vi "Valid waveforms Write.vi"(4 "error in (no error)":errorcluster, 5 "Value":T1[](array[typedef]), 6 "Container State":T4, 7 "Display State In":T2) -> (0 "error out":errorcluster, 3 "Display State Out":T2)   [LabVIEW 2020, in "Waveform (G3).xctl"]
uses:
  Waveform (G3).xctl
  <vilib>/_xctls/Container State.ctl
  State.ctl
  Utility VIs/Controls/KRing/KRing.xctl
  Tone (G3)/Tone (G3).xctl
  Noise (G3)/Noise (G3).xctl
  Noise (G3)/Noise (G3) - Persistent.ctl
  Waveform VIs/Waveform Enum (V3).ctl
  <vilib>/_xctls/XControlSupport.lvlib
panel:
  in  "Waveform":T1
  # "Replace the Value Control below with a Control of desired type.\nDo not remove this Control or the others from the connector pane.\nDo not change the connector pane pattern.\nThe Value control should always be the third terminal from top on the input side in the connector pane."
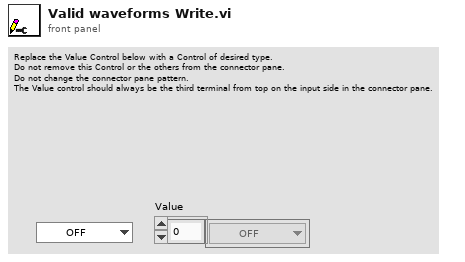
[diagram p1: front panel]
types:
  T1 = typedef "Waveform Enum (V3).ctl" = enum16{"OFF", "Tone", "Noise", "Pulse Train", "File", "FM Sweep", "Chirp Train", "Complex Tone", "FM Tone", "Vowel", "Ramp"}
  T2 = typedef "Waveform (G3).xctl/State.ctl" = cluster{"Waveform names":string[], "Valid":bool[], "enable menu":bool, "Controls":cluster{"Type ":refnum<vi>, "Tone ":refnum<vi>, "Noise":refnum<vi>}, "persistent":cluster{"noise":T3, "Sort":bool}, "multi":bool}
  T3 = typedef "Noise (G3).xctl/Noise (G3) - Persistent.ctl" = cluster{"Show Aweight":bool}
  T4 = typedef "XControlSupport.lvlib/Container State.ctl" = cluster{"Indicator?":bool, "Run Mode?":bool, " Refnum":refnum<vi>}
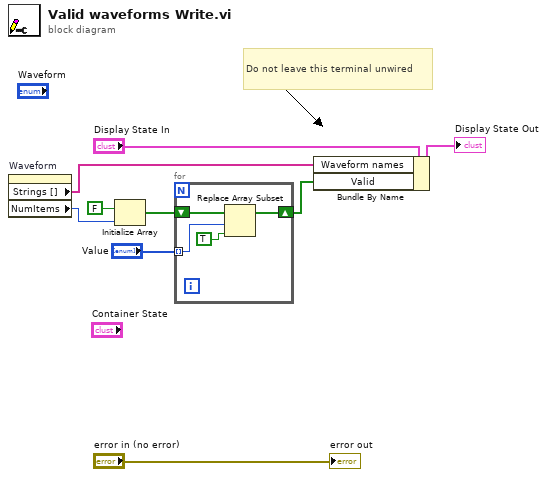
[diagram p0: block diagram]
diagram:
  # "Do not leave this terminal unwired"
  n1 = property on="Waveform" class="Enum (strict)"() -> ("Strings []"=w1:string[], "NumItems"=w2:u32)  [unwired: 2 in, 2 out]
  n2 = Initialize Array(FALSE, w2) -> (w6:bool[])
  n3 = for {
    shift-right: [w10] -> w3
    shift-left: w6 -> [w13]
    tunnel: "Value" -> [w12] mode=indexing
    n4 = Replace Array Subset(array=w13, new element=TRUE, index=w12) -> (w10:bool[])
  }
  n5 = Bundle By Name(cluster="Display State In", "Waveform names"=w1, "Valid"=w3) -> (→"Display State Out":T2)
  "error out" <- "error in (no error)"
